vi "Create.vi"(6 "Timeout ms (5000)":i32=5000, 8 "error in (no error)":errorcluster, 10 "VolatusAPI":refnum<class "VolatusAPI.lvclass">) -> (0 "error out":errorcluster, 3 "Historian API out":refnum<class "Historian API.lvclass">)   [LabVIEW 2020, in "VolatusHistorian.lvlib" / "Historian API.lvclass"]
uses:
  Historian API.lvclass
  Historian API.lvclass/Historian API.ctl
  Historian Identity/Historian Identity.lvclass
  Volatus/VolatusAPI/VolatusAPI.lvclass
  C:/dev/lv20CE/relink/lv-volatus/VolatusHistorian/Historian Identity/Historian Identity.lvclass
  C:/dev/lv20CE/relink/lv-volatus/Volatus/Identity/Identity.lvclass
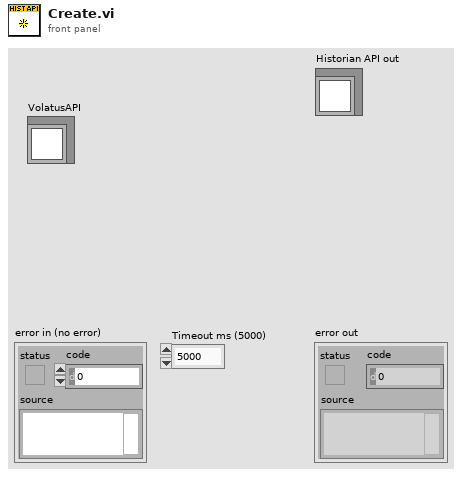
[diagram p1: front panel]
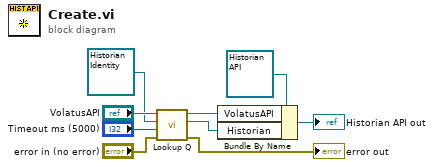
[diagram p0: block diagram]
diagram:
  n1 = call "Lookup Q.vi"("error in (no error)"="error in (no error)", "Timeout ms (0)"="Timeout ms (5000)", "Identity"=refnum<class "Historian Identity.lvclass"> refnum ("VolatusHistorian.lvlib:Historian Identity.lvclass"), "VolatusAPI in"="VolatusAPI") -> ("error out"=→"error out":errorcluster, "MessageQ"=w3:refnum<class "MessageQ.lvclass">, "VolatusAPI out"=w6:refnum<class "VolatusAPI.lvclass">)  [unwired: 5 in]
  n2 = Bundle By Name(cluster=refnum<class "Historian API.lvclass"> refnum ("Historian API in"), "VolatusAPI"=w6, "Historian"=w3) -> (→"Historian API out":refnum<class "Historian API.lvclass">)
